vi "Patern face 4.vi"(0 "Color Box 2":u32(colorbox), 1 "Color Box 3":u32(colorbox), 2 "Color Box 4":u32(colorbox), 3 "Color Box 5":u32(colorbox), 4 "Color Box 6":u32(colorbox), 5 "Color Box 7":u32(colorbox), 6 "Array":string[](array[string]), 7 "Color Box 8":u32(colorbox), 9 "Color Box 9":u32(colorbox), 11 "Color Box 10":u32(colorbox)) -> (15 "Final array":string[](array[string]))   [LabVIEW 2019]
panel:
  in  "?":bool
  # "FACE 3"
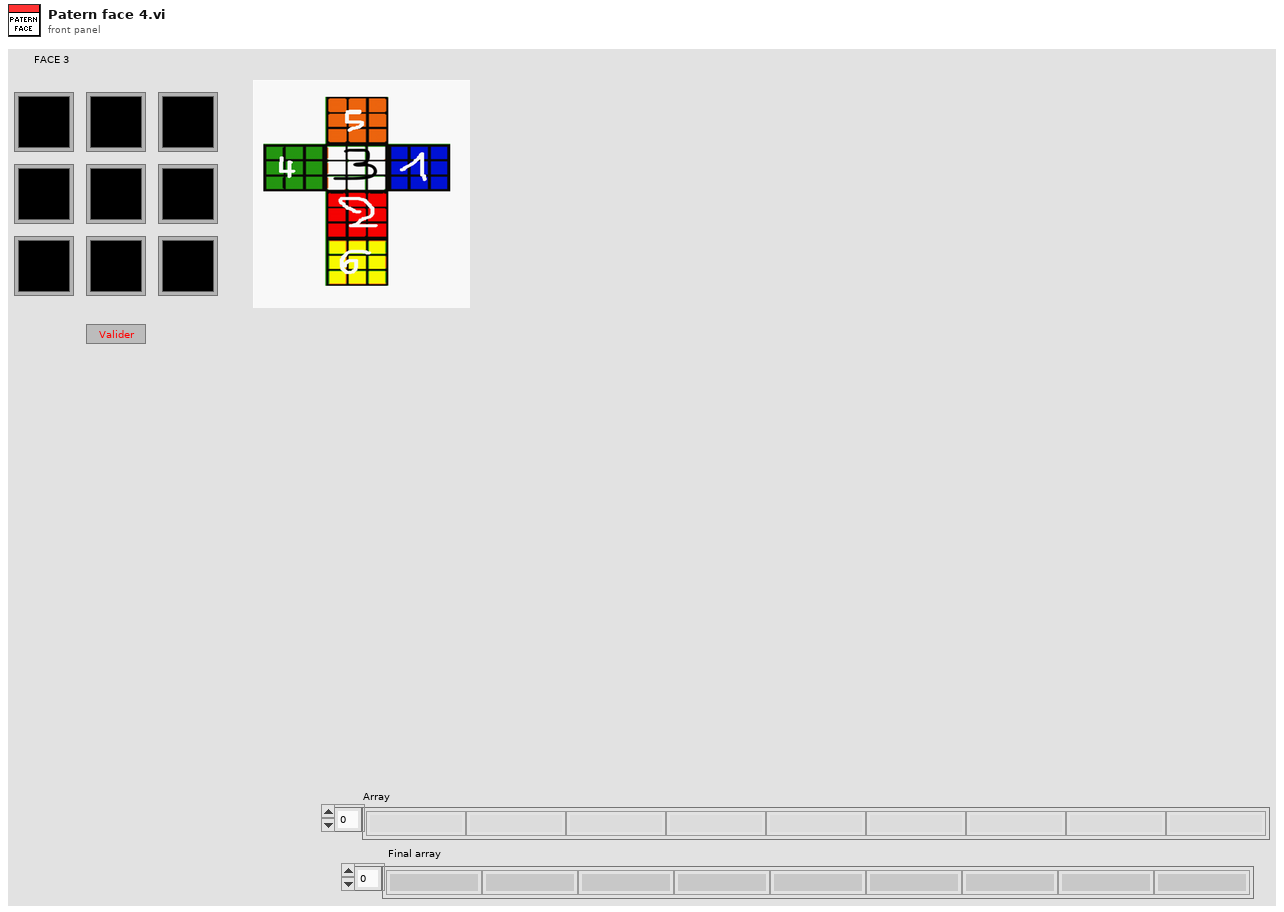
[diagram p1: front panel]
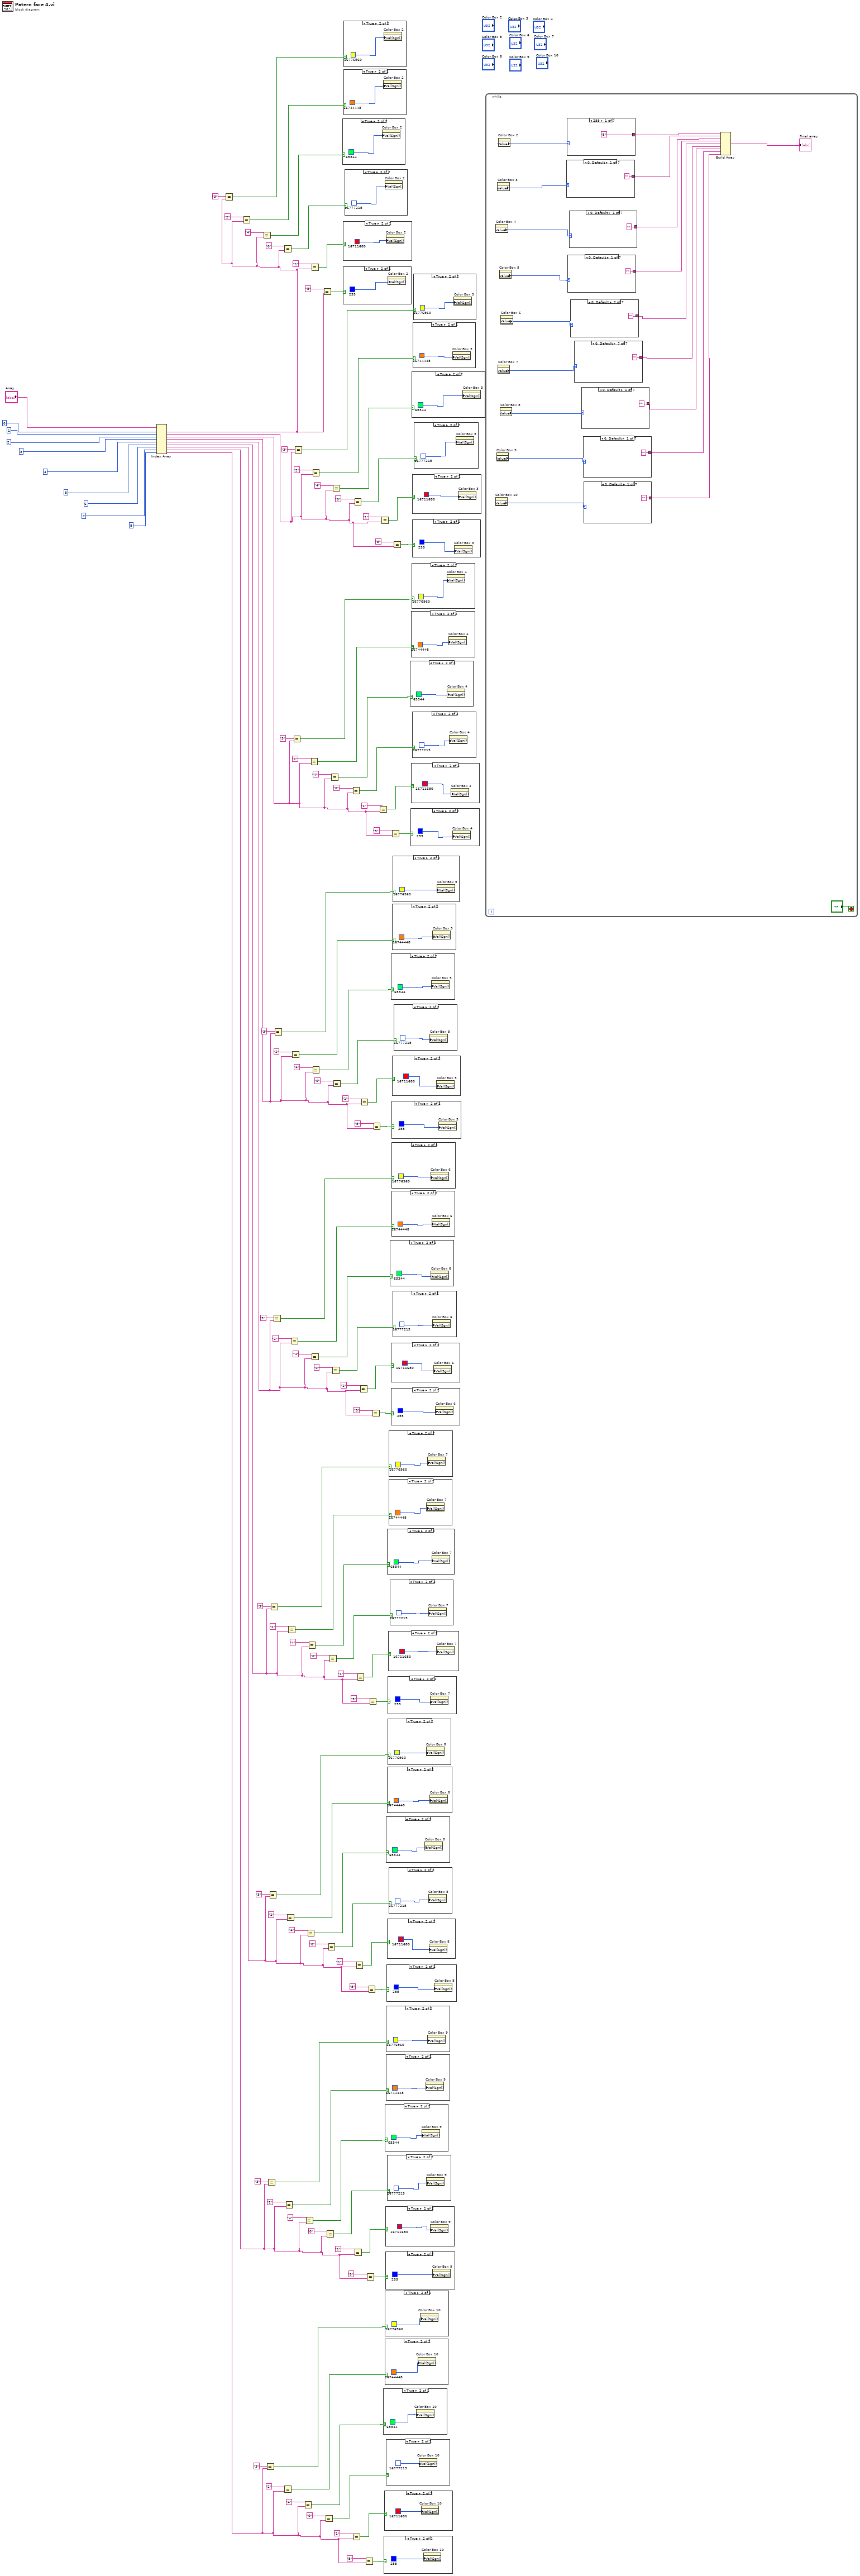
[diagram p0: block diagram]
diagram:
  n1 = Index Array(array="Array", index #1=0 ("index"), index #2=1 ("index (row)"), index #3=2 ("index (row)"), index #4=3 ("index (row)"), index #5=4 ("index (row)"), index #6=5 ("index (row)"), index #7=6 ("index (row)"), index #8=7 ("index (row)"), index #9=8 ("index")) -> (element #1=w106:string, element #2=w93:string, element #3=w79:string, element #4=w66:string, element #5=w53:string, element #6=w40:string, element #7=w27:string, element #8=w14:string, element #9=w1:string)
  n2 = Equal?(x="3", y=w106) -> (x = y?=w115:bool)
  n3 = Equal?(x="2", y=w106) -> (x = y?=w116:bool)
  n4 = Equal?(x="4", y=w106) -> (x = y?=w117:bool)
  n5 = Equal?(x="3", y=w1) -> (x = y?=w2:bool)
  n6 = Equal?(x="3", y=w14) -> (x = y?=w15:bool)
  n7 = Equal?(x="3", y=w27) -> (x = y?=w28:bool)
  n8 = Equal?(x="3", y=w40) -> (x = y?=w41:bool)
  n9 = Equal?(x="3", y=w53) -> (x = y?=w54:bool)
  n10 = Equal?(x="3", y=w66) -> (x = y?=w67:bool)
  n11 = Equal?(x="0", y=w106) -> (x = y?=w118:bool)
  n12 = Equal?(x="2", y=w1) -> (x = y?=w3:bool)
  n13 = Equal?(x="2", y=w14) -> (x = y?=w16:bool)
  n14 = Equal?(x="2", y=w27) -> (x = y?=w29:bool)
  n15 = Equal?(x="2", y=w40) -> (x = y?=w42:bool)
  n16 = Equal?(x="2", y=w53) -> (x = y?=w55:bool)
  n17 = Equal?(x="2", y=w66) -> (x = y?=w68:bool)
  n18 = Equal?(x="3", y=w79) -> (x = y?=w80:bool)
  n19 = Equal?(x="3", y=w93) -> (x = y?=w105:bool)
  n20 = Equal?(x="4", y=w1) -> (x = y?=w4:bool)
  n21 = Equal?(x="4", y=w14) -> (x = y?=w17:bool)
  n22 = Equal?(x="4", y=w27) -> (x = y?=w30:bool)
  n23 = Equal?(x="4", y=w40) -> (x = y?=w43:bool)
  n24 = Equal?(x="2", y=w79) -> (x = y?=w81:bool)
  n25 = Equal?(x="1", y=w106) -> (x = y?=w119:bool)
  n26 = Equal?(x="4", y=w53) -> (x = y?=w56:bool)
  n27 = Equal?(x="2", y=w93) -> (x = y?=w104:bool)
  n28 = Equal?(x="4", y=w66) -> (x = y?=w69:bool)
  n29 = Equal?(x="5", y=w106) -> (x = y?=w127:bool)
  n30 = Equal?(x="0", y=w1) -> (x = y?=w5:bool)
  n31 = Equal?(x="0", y=w14) -> (x = y?=w18:bool)
  n32 = Equal?(x="0", y=w27) -> (x = y?=w31:bool)
  n33 = Equal?(x="0", y=w40) -> (x = y?=w44:bool)
  n34 = Equal?(x="4", y=w79) -> (x = y?=w82:bool)
  n35 = Equal?(x="0", y=w53) -> (x = y?=w57:bool)
  n36 = Equal?(x="4", y=w93) -> (x = y?=w103:bool)
  n37 = Equal?(x="0", y=w66) -> (x = y?=w70:bool)
  n38 = case shown="True" w117 {
    frame False {
    }
    frame True {
      n39 = property on="Color Box 2" class="ColBox"("Val(Sgnl)"=u32 65344 ("Color Box 2")) -> ()  [unwired: 2 in, 2 out]
    }
  }
  n40 = case shown="True" w127 {
    frame False {
    }
    frame True {
      n41 = property on="Color Box 2" class="ColBox"("Val(Sgnl)"=u32 255 ("Color Box 2")) -> ()  [unwired: 2 in, 2 out]
    }
  }
  n42 = case shown="True" w119 {
    frame False {
    }
    frame True {
      n43 = property on="Color Box 2" class="ColBox"("Val(Sgnl)"=u32 16711680 ("Color Box 2")) -> ()  [unwired: 2 in, 2 out]
    }
  }
  n44 = case shown="True" w116 {
    frame False {
    }
    frame True {
      n45 = property on="Color Box 2" class="ColBox"("Val(Sgnl)"=u32 16744448 ("Color Box 2")) -> ()  [unwired: 2 in, 2 out]
    }
  }
  n46 = case shown="True" w115 {
    frame False {
    }
    frame True {
      n47 = property on="Color Box 2" class="ColBox"("Val(Sgnl)"=u32 16776960 ("Color Box 2")) -> ()  [unwired: 2 in, 2 out]
    }
  }
  n48 = case shown="True" w118 {
    frame False {
    }
    frame True {
      n49 = property on="Color Box 2" class="ColBox"("Val(Sgnl)"=u32 16777215 ("Color Box 2")) -> ()  [unwired: 2 in, 2 out]
    }
  }
  n50 = Equal?(x="0", y=w79) -> (x = y?=w83:bool)
  n51 = Equal?(x="1", y=w1) -> (x = y?=w6:bool)
  n52 = Equal?(x="0", y=w93) -> (x = y?=w102:bool)
  n53 = Equal?(x="1", y=w14) -> (x = y?=w19:bool)
  n54 = Equal?(x="1", y=w27) -> (x = y?=w32:bool)
  n55 = Equal?(x="1", y=w40) -> (x = y?=w45:bool)
  n56 = Equal?(x="1", y=w53) -> (x = y?=w58:bool)
  n57 = Equal?(x="1", y=w66) -> (x = y?=w71:bool)
  n58 = Equal?(x="5", y=w1) -> (x = y?=w13:bool)
  n59 = Equal?(x="5", y=w14) -> (x = y?=w26:bool)
  n60 = Equal?(x="5", y=w27) -> (x = y?=w39:bool)
  n61 = Equal?(x="5", y=w40) -> (x = y?=w52:bool)
  n62 = Equal?(x="5", y=w53) -> (x = y?=w65:bool)
  n63 = Equal?(x="5", y=w66) -> (x = y?=w78:bool)
  n64 = Equal?(x="1", y=w79) -> (x = y?=w84:bool)
  n65 = Equal?(x="1", y=w93) -> (x = y?=w101:bool)
  n66 = case shown="True" w4 {
    frame False {
    }
    frame True {
      n67 = property on="Color Box 10" class="ColBox"("Val(Sgnl)"=u32 65344 ("Color Box 2")) -> ()  [unwired: 2 in, 2 out]
    }
  }
  n68 = case shown="True" w13 {
    frame False {
    }
    frame True {
      n69 = property on="Color Box 10" class="ColBox"("Val(Sgnl)"=u32 255 ("Color Box 2")) -> ()  [unwired: 2 in, 2 out]
    }
  }
  n70 = case shown="True" w6 {
    frame False {
    }
    frame True {
      n71 = property on="Color Box 10" class="ColBox"("Val(Sgnl)"=u32 16711680 ("Color Box 2")) -> ()  [unwired: 2 in, 2 out]
    }
  }
  n72 = case shown="True" w17 {
    frame False {
    }
    frame True {
      n73 = property on="Color Box 9" class="ColBox"("Val(Sgnl)"=u32 65344 ("Color Box 2")) -> ()  [unwired: 2 in, 2 out]
    }
  }
  n74 = case shown="True" w3 {
    frame False {
    }
    frame True {
      n75 = property on="Color Box 10" class="ColBox"("Val(Sgnl)"=u32 16744448 ("Color Box 2")) -> ()  [unwired: 2 in, 2 out]
    }
  }
  n76 = case shown="True" w2 {
    frame False {
    }
    frame True {
      n77 = property on="Color Box 10" class="ColBox"("Val(Sgnl)"=u32 16776960 ("Color Box 2")) -> ()  [unwired: 2 in, 2 out]
    }
  }
  n78 = case shown="True" w26 {
    frame False {
    }
    frame True {
      n79 = property on="Color Box 9" class="ColBox"("Val(Sgnl)"=u32 255 ("Color Box 2")) -> ()  [unwired: 2 in, 2 out]
    }
  }
  n80 = case shown="True" w19 {
    frame False {
    }
    frame True {
      n81 = property on="Color Box 9" class="ColBox"("Val(Sgnl)"=u32 16711680 ("Color Box 2")) -> ()  [unwired: 2 in, 2 out]
    }
  }
  n82 = case shown="True" w30 {
    frame False {
    }
    frame True {
      n83 = property on="Color Box 8" class="ColBox"("Val(Sgnl)"=u32 65344 ("Color Box 2")) -> ()  [unwired: 2 in, 2 out]
    }
  }
  n84 = case shown="True" w16 {
    frame False {
    }
    frame True {
      n85 = property on="Color Box 9" class="ColBox"("Val(Sgnl)"=u32 16744448 ("Color Box 2")) -> ()  [unwired: 2 in, 2 out]
    }
  }
  n86 = case shown="True" w5 {
    frame False {
    }
    frame True {
      n87 = property on="Color Box 10" class="ColBox"("Val(Sgnl)"=u32 16777215 ("Color Box 2")) -> ()  [unwired: 2 in, 2 out]
    }
  }
  n88 = case shown="True" w15 {
    frame False {
    }
    frame True {
      n89 = property on="Color Box 9" class="ColBox"("Val(Sgnl)"=u32 16776960 ("Color Box 2")) -> ()  [unwired: 2 in, 2 out]
    }
  }
  n90 = case shown="True" w39 {
    frame False {
    }
    frame True {
      n91 = property on="Color Box 8" class="ColBox"("Val(Sgnl)"=u32 255 ("Color Box 2")) -> ()  [unwired: 2 in, 2 out]
    }
  }
  n92 = case shown="True" w32 {
    frame False {
    }
    frame True {
      n93 = property on="Color Box 8" class="ColBox"("Val(Sgnl)"=u32 16711680 ("Color Box 2")) -> ()  [unwired: 2 in, 2 out]
    }
  }
  n94 = case shown="True" w43 {
    frame False {
    }
    frame True {
      n95 = property on="Color Box 7" class="ColBox"("Val(Sgnl)"=u32 65344 ("Color Box 2")) -> ()  [unwired: 2 in, 2 out]
    }
  }
  n96 = case shown="True" w29 {
    frame False {
    }
    frame True {
      n97 = property on="Color Box 8" class="ColBox"("Val(Sgnl)"=u32 16744448 ("Color Box 2")) -> ()  [unwired: 2 in, 2 out]
    }
  }
  n98 = case shown="True" w18 {
    frame False {
    }
    frame True {
      n99 = property on="Color Box 9" class="ColBox"("Val(Sgnl)"=u32 16777215 ("Color Box 2")) -> ()  [unwired: 2 in, 2 out]
    }
  }
  n100 = case shown="True" w28 {
    frame False {
    }
    frame True {
      n101 = property on="Color Box 8" class="ColBox"("Val(Sgnl)"=u32 16776960 ("Color Box 2")) -> ()  [unwired: 2 in, 2 out]
    }
  }
  n102 = case shown="True" w52 {
    frame False {
    }
    frame True {
      n103 = property on="Color Box 7" class="ColBox"("Val(Sgnl)"=u32 255 ("Color Box 2")) -> ()  [unwired: 2 in, 2 out]
    }
  }
  n104 = case shown="True" w45 {
    frame False {
    }
    frame True {
      n105 = property on="Color Box 7" class="ColBox"("Val(Sgnl)"=u32 16711680 ("Color Box 2")) -> ()  [unwired: 2 in, 2 out]
    }
  }
  n106 = case shown="True" w42 {
    frame False {
    }
    frame True {
      n107 = property on="Color Box 7" class="ColBox"("Val(Sgnl)"=u32 16744448 ("Color Box 2")) -> ()  [unwired: 2 in, 2 out]
    }
  }
  n108 = case shown="True" w31 {
    frame False {
    }
    frame True {
      n109 = property on="Color Box 8" class="ColBox"("Val(Sgnl)"=u32 16777215 ("Color Box 2")) -> ()  [unwired: 2 in, 2 out]
    }
  }
  n110 = case shown="True" w41 {
    frame False {
    }
    frame True {
      n111 = property on="Color Box 7" class="ColBox"("Val(Sgnl)"=u32 16776960 ("Color Box 2")) -> ()  [unwired: 2 in, 2 out]
    }
  }
  n112 = case shown="True" w44 {
    frame False {
    }
    frame True {
      n113 = property on="Color Box 7" class="ColBox"("Val(Sgnl)"=u32 16777215 ("Color Box 2")) -> ()  [unwired: 2 in, 2 out]
    }
  }
  n114 = case shown="True" w56 {
    frame False {
    }
    frame True {
      n115 = property on="Color Box 6" class="ColBox"("Val(Sgnl)"=u32 65344 ("Color Box 2")) -> ()  [unwired: 2 in, 2 out]
    }
  }
  n116 = Equal?(x="5", y=w79) -> (x = y?=w91:bool)
  n117 = case shown="True" w65 {
    frame False {
    }
    frame True {
      n118 = property on="Color Box 6" class="ColBox"("Val(Sgnl)"=u32 255 ("Color Box 2")) -> ()  [unwired: 2 in, 2 out]
    }
  }
  n119 = case shown="True" w69 {
    frame False {
    }
    frame True {
      n120 = property on="Color Box 5" class="ColBox"("Val(Sgnl)"=u32 65344 ("Color Box 2")) -> ()  [unwired: 2 in, 2 out]
    }
  }
  n121 = case shown="True" w58 {
    frame False {
    }
    frame True {
      n122 = property on="Color Box 6" class="ColBox"("Val(Sgnl)"=u32 16711680 ("Color Box 2")) -> ()  [unwired: 2 in, 2 out]
    }
  }
  n123 = case shown="True" w55 {
    frame False {
    }
    frame True {
      n124 = property on="Color Box 6" class="ColBox"("Val(Sgnl)"=u32 16744448 ("Color Box 2")) -> ()  [unwired: 2 in, 2 out]
    }
  }
  n125 = case shown="True" w78 {
    frame False {
    }
    frame True {
      n126 = property on="Color Box 5" class="ColBox"("Val(Sgnl)"=u32 255 ("Color Box 2")) -> ()  [unwired: 2 in, 2 out]
    }
  }
  n127 = case shown="True" w54 {
    frame False {
    }
    frame True {
      n128 = property on="Color Box 6" class="ColBox"("Val(Sgnl)"=u32 16776960 ("Color Box 2")) -> ()  [unwired: 2 in, 2 out]
    }
  }
  n129 = Equal?(x="5", y=w93) -> (x = y?=w94:bool)
  n130 = case shown="True" w71 {
    frame False {
    }
    frame True {
      n131 = property on="Color Box 5" class="ColBox"("Val(Sgnl)"=u32 16711680 ("Color Box 2")) -> ()  [unwired: 2 in, 2 out]
    }
  }
  n132 = case shown="True" w68 {
    frame False {
    }
    frame True {
      n133 = property on="Color Box 5" class="ColBox"("Val(Sgnl)"=u32 16744448 ("Color Box 2")) -> ()  [unwired: 2 in, 2 out]
    }
  }
  n134 = case shown="True" w67 {
    frame False {
    }
    frame True {
      n135 = property on="Color Box 5" class="ColBox"("Val(Sgnl)"=u32 16776960 ("Color Box 2")) -> ()  [unwired: 2 in, 2 out]
    }
  }
  n136 = case shown="True" w57 {
    frame False {
    }
    frame True {
      n137 = property on="Color Box 6" class="ColBox"("Val(Sgnl)"=u32 16777215 ("Color Box 2")) -> ()  [unwired: 2 in, 2 out]
    }
  }
  n138 = case shown="True" w70 {
    frame False {
    }
    frame True {
      n139 = property on="Color Box 5" class="ColBox"("Val(Sgnl)"=u32 16777215 ("Color Box 2")) -> ()  [unwired: 2 in, 2 out]
    }
  }
  n140 = case shown="True" w82 {
    frame False {
    }
    frame True {
      n141 = property on="Color Box 4" class="ColBox"("Val(Sgnl)"=u32 65344 ("Color Box 2")) -> ()  [unwired: 2 in, 2 out]
    }
  }
  n142 = case shown="True" w91 {
    frame False {
    }
    frame True {
      n143 = property on="Color Box 4" class="ColBox"("Val(Sgnl)"=u32 255 ("Color Box 2")) -> ()  [unwired: 2 in, 2 out]
    }
  }
  n144 = case shown="True" w84 {
    frame False {
    }
    frame True {
      n145 = property on="Color Box 4" class="ColBox"("Val(Sgnl)"=u32 16711680 ("Color Box 2")) -> ()  [unwired: 2 in, 2 out]
    }
  }
  n146 = case shown="True" w81 {
    frame False {
    }
    frame True {
      n147 = property on="Color Box 4" class="ColBox"("Val(Sgnl)"=u32 16744448 ("Color Box 2")) -> ()  [unwired: 2 in, 2 out]
    }
  }
  n148 = case shown="True" w103 {
    frame False {
    }
    frame True {
      n149 = property on="Color Box 3" class="ColBox"("Val(Sgnl)"=u32 65344 ("Color Box 2")) -> ()  [unwired: 2 in, 2 out]
    }
  }
  n150 = case shown="True" w80 {
    frame False {
    }
    frame True {
      n151 = property on="Color Box 4" class="ColBox"("Val(Sgnl)"=u32 16776960 ("Color Box 2")) -> ()  [unwired: 2 in, 2 out]
    }
  }
  n152 = case shown="True" w94 {
    frame False {
    }
    frame True {
      n153 = property on="Color Box 3" class="ColBox"("Val(Sgnl)"=u32 255 ("Color Box 2")) -> ()  [unwired: 2 in, 2 out]
    }
  }
  n154 = case shown="True" w101 {
    frame False {
    }
    frame True {
      n155 = property on="Color Box 3" class="ColBox"("Val(Sgnl)"=u32 16711680 ("Color Box 2")) -> ()  [unwired: 2 in, 2 out]
    }
  }
  n156 = case shown="True" w83 {
    frame False {
    }
    frame True {
      n157 = property on="Color Box 4" class="ColBox"("Val(Sgnl)"=u32 16777215 ("Color Box 2")) -> ()  [unwired: 2 in, 2 out]
    }
  }
  n158 = case shown="True" w104 {
    frame False {
    }
    frame True {
      n159 = property on="Color Box 3" class="ColBox"("Val(Sgnl)"=u32 16744448 ("Color Box 2")) -> ()  [unwired: 2 in, 2 out]
    }
  }
  n160 = case shown="True" w105 {
    frame False {
    }
    frame True {
      n161 = property on="Color Box 3" class="ColBox"("Val(Sgnl)"=u32 16776960 ("Color Box 2")) -> ()  [unwired: 2 in, 2 out]
    }
  }
  n162 = case shown="True" w102 {
    frame False {
    }
    frame True {
      n163 = property on="Color Box 3" class="ColBox"("Val(Sgnl)"=u32 16777215 ("Color Box 2")) -> ()  [unwired: 2 in, 2 out]
    }
  }
  n164 = while {
    stop <- "?" stop-if-true
    n165 = property on="Color Box 10" class="ColBox"() -> ("Value"=w192:u32)  [unwired: 2 in, 2 out]
    n166 = property on="Color Box 4" class="ColBox"() -> ("Value"=w198:u32)  [unwired: 2 in, 2 out]
    n167 = property on="Color Box 9" class="ColBox"() -> ("Value"=w193:u32)  [unwired: 2 in, 2 out]
    n168 = property on="Color Box 3" class="ColBox"() -> ("Value"=w182:u32)  [unwired: 2 in, 2 out]
    n169 = property on="Color Box 7" class="ColBox"() -> ("Value"=w195:u32)  [unwired: 2 in, 2 out]
    n170 = property on="Color Box 2" class="ColBox"() -> ("Value"=w183:u32)  [unwired: 2 in, 2 out]
    n171 = property on="Color Box 5" class="ColBox"() -> ("Value"=w197:u32)  [unwired: 2 in, 2 out]
    n172 = property on="Color Box 8" class="ColBox"() -> ("Value"=w194:u32)  [unwired: 2 in, 2 out]
    n173 = property on="Color Box 6" class="ColBox"() -> ("Value"=w196:u32)  [unwired: 2 in, 2 out]
    n174 = case shown="0, Default" w182 {
      tunnel: ["" "5" "1" "0" "4" "2" "3"] -> w199
      frame 0, Default {
      }
      frame 255 {
      }
      frame 16711680 {
      }
      frame 16777215 {
      }
      frame 65344 {
      }
      frame 16744448 {
      }
      frame 16776960 {
      }
    }
    n175 = case shown="255" w183 {
      tunnel: ["5" "1" "0" "4" "2" "3" ""] -> w200
      frame 255 {
      }
      frame 16711680 {
      }
      frame 16777215 {
      }
      frame 65344 {
      }
      frame 16744448 {
      }
      frame 16776960 {
      }
      frame 0, Default {
      }
    }
    n176 = case shown="0, Default" w197 {
      tunnel: ["" "5" "1" "0" "4" "2" "3"] -> w190
      frame 0, Default {
      }
      frame 255 {
      }
      frame 16711680 {
      }
      frame 16777215 {
      }
      frame 65344 {
      }
      frame 16744448 {
      }
      frame 16776960 {
      }
    }
    n177 = case shown="0, Default" w198 {
      tunnel: ["" "5" "1" "0" "4" "2" "3"] -> w191
      frame 0, Default {
      }
      frame 255 {
      }
      frame 16711680 {
      }
      frame 16777215 {
      }
      frame 65344 {
      }
      frame 16744448 {
      }
      frame 16776960 {
      }
    }
    n178 = case shown="0, Default" w196 {
      tunnel: ["5" "1" "0" "4" "2" "3" ""] -> w189
      frame 255 {
      }
      frame 16711680 {
      }
      frame 16777215 {
      }
      frame 65344 {
      }
      frame 16744448 {
      }
      frame 16776960 {
      }
      frame 0, Default {
      }
    }
    n179 = case shown="0, Default" w195 {
      tunnel: ["5" "1" "0" "4" "2" "3" ""] -> w188
      frame 255 {
      }
      frame 16711680 {
      }
      frame 16777215 {
      }
      frame 65344 {
      }
      frame 16744448 {
      }
      frame 16776960 {
      }
      frame 0, Default {
      }
    }
    n180 = case shown="0, Default" w194 {
      tunnel: ["" "5" "1" "0" "4" "2" "3"] -> w187
      frame 0, Default {
      }
      frame 255 {
      }
      frame 16711680 {
      }
      frame 16777215 {
      }
      frame 65344 {
      }
      frame 16744448 {
      }
      frame 16776960 {
      }
    }
    n181 = case shown="0, Default" w193 {
      tunnel: ["" "5" "1" "0" "4" "2" "3"] -> w186
      frame 0, Default {
      }
      frame 255 {
      }
      frame 16711680 {
      }
      frame 16777215 {
      }
      frame 65344 {
      }
      frame 16744448 {
      }
      frame 16776960 {
      }
    }
    n182 = case shown="0, Default" w192 {
      tunnel: ["" "5" "1" "0" "4" "2" "3"] -> w185
      frame 0, Default {
      }
      frame 255 {
      }
      frame 16711680 {
      }
      frame 16777215 {
      }
      frame 65344 {
      }
      frame 16744448 {
      }
      frame 16776960 {
      }
    }
    n183 = Build Array(w200, w199, w191, w190, w189, w188, w187, w186, w185) -> (→"Final array":string[])
  }
